vi "Init Log Text File Sink.vi"(8 "error in (no error)":errorcluster, 11 "Text File Sink in":refnum<class "Text File Sink.lvclass">) -> (0 "error out":errorcluster, 3 "Text File Sink out":refnum<class "Text File Sink.lvclass">)   [LabVIEW 2016, in "Stream Log.lvlib" / "Text File Sink.lvclass"]
doc: "--\nCopyright © 2017 Composed SystemsI All rights reserved.\n\nAuthor: Jon McBee <jon.mcbee@composed.io>\n\nThis library is provided \"AS IS\" ,WITHOUT WARRANTIES OR\nCONDITIONS OF ANY KIND, either express or implied.\n\nComposed Systems -- composed.io\n\nStream 0.0.1.1\nJon McBee - Composed Systems\nCopyright (c) 2017, Composed Systems"
uses:
  <userlib>/Composed Systems/Stream/Log/Text File Sink/Text File Sink.lvclass
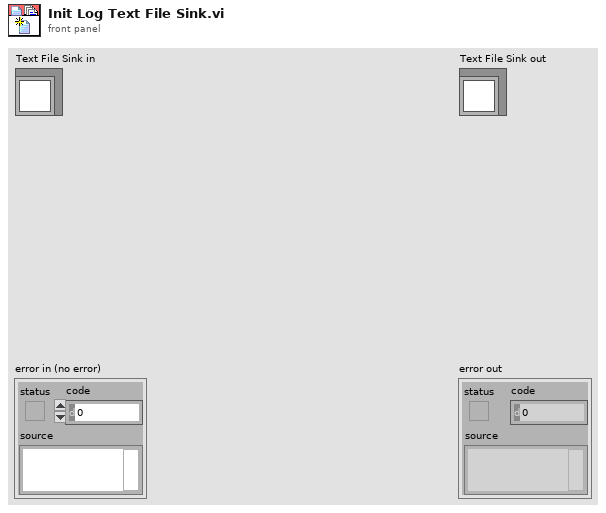
[diagram p1: front panel]
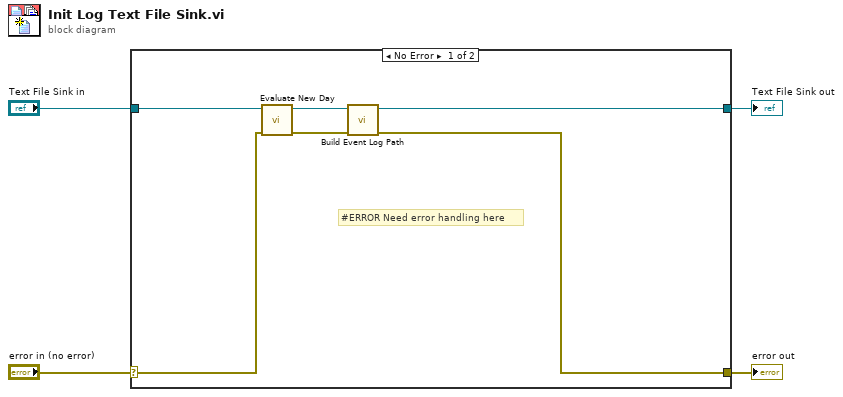
[diagram p0: block diagram]
diagram:
  n1 = case shown="No Error" "error in (no error)" {
    selector: "error in (no error)" -> [w6 w12]
    tunnel: [w5 w12] -> w3
    tunnel: [w8 w11] -> w1
    tunnel: "Text File Sink in" -> [w10 w11]
    frame No Error {
      # "#ERROR Need error handling here"
      n2 = call <userlib>:"Evaluate New Day.vi"("error in (no error)"=w6, "Text File Sink in"=w10) -> ("error out"=w7:errorcluster, "Text File Sink out"=w9:refnum<class "Text File Sink.lvclass">)  [unwired: 8 in]
      n3 = call <userlib>:"Build Event Log Path.vi"("error in (no error)"=w7, "Text File Sink in"=w9) -> ("error out"=w5:errorcluster, "Text File Sink out"=w8:refnum<class "Text File Sink.lvclass">)  [unwired: 8 in]
    }
    frame Error {
    }
  }
  "error out" <- w3
  "Text File Sink out" <- w1
